vi "FRCts20_WebMethods_Redirect_Request.vi"(7 "response code (200)":i32(ring)=200 items=["100"=100, "101"=101, "200"=200, "201"=201, "202"=202, "203"=203, "204"=204, "205"=205, "206"=206, "300"=300, "301"=301, "302"=302, "303"=303, "304"=304, "305"=305, "306"=306, "307"=307, "400"=400, "401"=401, "402"=402, "403"=403, "404"=404, "405"=405, "406"=406, "407"=407, "408"=408, "409"=409, "410"=410, "411"=411, "412"=412, "413"=413, "414"=414, "415"=415, "416"=416, "417"=417, "500"=500, "501"=501, "502"=502, "503"=503, "504"=504, "505"=505], 8 "error in (no error)":errorcluster, 10 "Request":u32, 11 "httpRequestID":u32) -> (0 "error out":errorcluster, 3 "httpRequestID out":u32)   [LabVIEW 2014, in "FRCts20_WebMethods.lvlib"]
uses:
  FRCts20_WebMethods.lvlib
  <vilib>/wsapi/NI_WebServices.lvlib
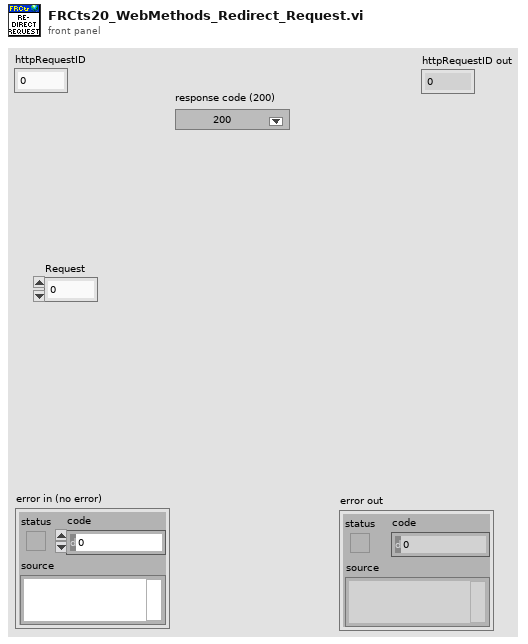
[diagram p1: front panel]
types:
  T1 = typedef "FRCts20_WebMethods.lvlib/FRCts20_WebMethods_ctl_returntype.ctl" = string
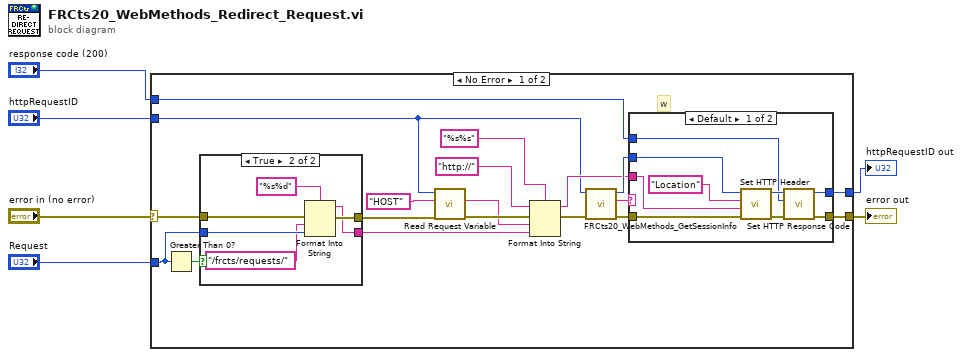
[diagram p0: block diagram]
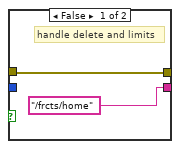
[diagram p2: hidden frame]
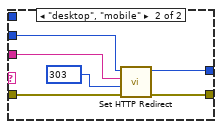
[diagram p3: hidden frame]
diagram:
  n1 = case shown="No Error" "error in (no error)" {
    selector: "error in (no error)" -> [w9 w49]
    tunnel: [w18 w49] -> w6
    tunnel: "httpRequestID" -> [w11 w50]
    tunnel: [w17 w50] -> w3
    tunnel: "response code (200)" -> [w15 _]
    tunnel: "Request" -> [w7 _]
    frame No Error {
      # "w"
      n2 = Greater Than 0?(x=w7) -> (x > 0?=w10:bool)
      n3 = case shown="True" w10 {
        tunnel: ["/frcts/home" w30] -> w23
        tunnel: [w26 w33] -> w8
        tunnel: w9 -> [w26 w32]
        tunnel: w7 -> [_ w29]
        frame False {
          # "handle delete and limits"
        }
        frame True {
          n4 = Format Into String(format string="%s%d", error in=w32, "/frcts/requests/", w29) -> (resulting string=w30:string, error out=w33:errorcluster)  [unwired: 1 in]
        }
      }
      n5 = call <vilib>:"Read Request Variable.vi"("error in (no error)"=w8, "variable name"="HOST", "httpRequestID"=w11) -> ("error out"=w14:errorcluster, "value"=w13:string)  [unwired: 6 in, 1 out]
      n6 = Format Into String(format string="%s%s", initial string="http://", error in=w14, w13, w23) -> (resulting string=w16:string, error out=w19:errorcluster)
      n7 = call "FRCts20_WebMethods_GetSessionInfo.vi"("error in"=w19, "httpRequestID"=w11) -> ("error out"=w21:errorcluster, "Return Type"=w22:T1, "httpRequestID out"=w20:u32)  [unwired: 7 in]
      n8 = case shown="Default" w22 {
        tunnel: [w38 w48] -> w18
        tunnel: [w35 w47] -> w17
        tunnel: w21 -> [w42 w45]
        tunnel: w20 -> [w41 w44]
        tunnel: w16 -> [w39 w43]
        tunnel: w15 -> [w34 _]
        frame Default {
          n9 = call <vilib>:"Set HTTP Header.vi"("error in (no error)"=w42, "header value"=w39, "header"="Location", "httpRequestID"=w41) -> ("error out"=w37:errorcluster, "httpRequestID out"=w36:u32)  [unwired: 6 in]
          n10 = call <vilib>:"Set HTTP Response Code.vi"("error in (no error)"=w37, "response code (200)"=w34, "httpRequestID"=w36) -> ("error out"=w38:errorcluster, "httpRequestID out"=w35:u32)  [unwired: 7 in]
        }
        frame "desktop", "mobile" {
          w46 = 303 items=["100"=100, "101"=101, "200"=200, "201"=201, "202"=202, "203"=203, "204"=204, "205"=205, "206"=206, "300"=300, "301"=301, "302"=302, "303"=303, "304"=304, "305"=305, "306"=306, "307"=307, "400"=400, "401"=401, "402"=402, "403"=403, "404"=404, "405"=405, "406"=406, "407"=407, "408"=408, "409"=409, "410"=410, "411"=411, "412"=412, "413"=413, "414"=414, "415"=415, "416"=416, "417"=417, "500"=500, "501"=501, "502"=502, "503"=503, "504"=504, "505"=505] ("response code (307)")
          n11 = call <vilib>:"Set HTTP Redirect.vi"("error in (no error)"=w45, "response code (307)"=w46, "redirect URL"=w43, "httpRequestID"=w44) -> ("error out"=w48:errorcluster, "httpRequestID out"=w47:u32)  [unwired: 6 in]
        }
      }
    }
    frame Error {
    }
  }
  "error out" <- w6
  "httpRequestID out" <- w3
